vi "FAMM-FixPath.vi"(6 "path-IN":path, 8 "error in (no error)":errorcluster, 11 "FAMM in":T1={"FAMM_PAQ_Layers"=0, "FAMM_PAQ_resolution"=0.0, "PAQ_TAGs"=[], "WAQ_TAGs"=[], "EAQ_TAGs"=[], "All_TAGs"=[], "PAQtagProps"=[], "WAQtagProps"=[], "EAQtagProps"=[], "DBAL_class"=refnum, "PAQ_memory"=[], "PAQupdates"=[], "FAMM_Size"={"other"=0, "1day"=0, "1week"=0}, "DatabaseFileExtention"="", "DatabaseSaveRate"=0.0, "Database_path"=path "G:/Sgraph_database", "DBAL-Queue"=refnum, "OS_name"="undefined"} {"FAMM_Size"."1week" format="%.0p"; "FAMM_Size"."1day" format="%.0p"; "FAMM_Size"."other" format="%.0p"; "EAQtagProps"."TagFunc" format="%08x"; "EAQtagProps"."RangeL" format="%.2f"; "EAQtagProps"."RangeH" format="%.2f"; "WAQtagProps"."TagFunc" format="%08x"; "WAQtagProps"."RangeL" format="%.2f"; "WAQtagProps"."RangeH" format="%.2f"; "PAQtagProps"."TagFunc" format="%08x"; "PAQtagProps"."RangeL" format="%.2f"; "PAQtagProps"."RangeH" format="%.2f"; "FAMM_PAQ_resolution" format="%.1p"}) -> (0 "error out":errorcluster, 3 "FAMM out":T1={"FAMM_PAQ_Layers"=0, "FAMM_PAQ_resolution"=0.0, "PAQ_TAGs"=[], "WAQ_TAGs"=[], "EAQ_TAGs"=[], "All_TAGs"=[], "PAQtagProps"=[], "WAQtagProps"=[], "EAQtagProps"=[], "DBAL_class"=refnum, "PAQ_memory"=[], "PAQupdates"=[], "FAMM_Size"={"other"=0, "1day"=0, "1week"=0}, "DatabaseFileExtention"="", "DatabaseSaveRate"=0.0, "Database_path"=path "G:/Sgraph_database", "DBAL-Queue"=refnum, "OS_name"="undefined"} {"FAMM_Size"."1week" format="%.0p"; "FAMM_Size"."1day" format="%.0p"; "FAMM_Size"."other" format="%.0p"; "EAQtagProps"."TagFunc" format="%08x"; "EAQtagProps"."RangeL" format="%.2f"; "EAQtagProps"."RangeH" format="%.2f"; "WAQtagProps"."TagFunc" format="%08x"; "WAQtagProps"."RangeL" format="%.2f"; "WAQtagProps"."RangeH" format="%.2f"; "PAQtagProps"."TagFunc" format="%08x"; "PAQtagProps"."RangeL" format="%.2f"; "PAQtagProps"."RangeH" format="%.2f"; "FAMM_PAQ_resolution" format="%.1p"}, 4 "path-OUT":path)   [LabVIEW 2020, in "Sgraph_lib_V1.lvlib" / "FAMM.lvclass"]
doc: "Fix the OS dependency of a file path.\nUnix path definitions (Mac and Linux) differ from Windows type path definitions and therefore need to be adapted."
uses:
  FAMM.lvclass
  controls/FAMM-attributes.ctl
  Common/controls/typedef_com_TagProp.ctl
  DBAL/DBAL.lvclass
  PAQ-memory.lvclass
  DBAL/controls/DBAL_Command.ctl
  DBAL/controls/DBAL-commands.ctl
  Builds/Sgraph_lib_V1.lvlib
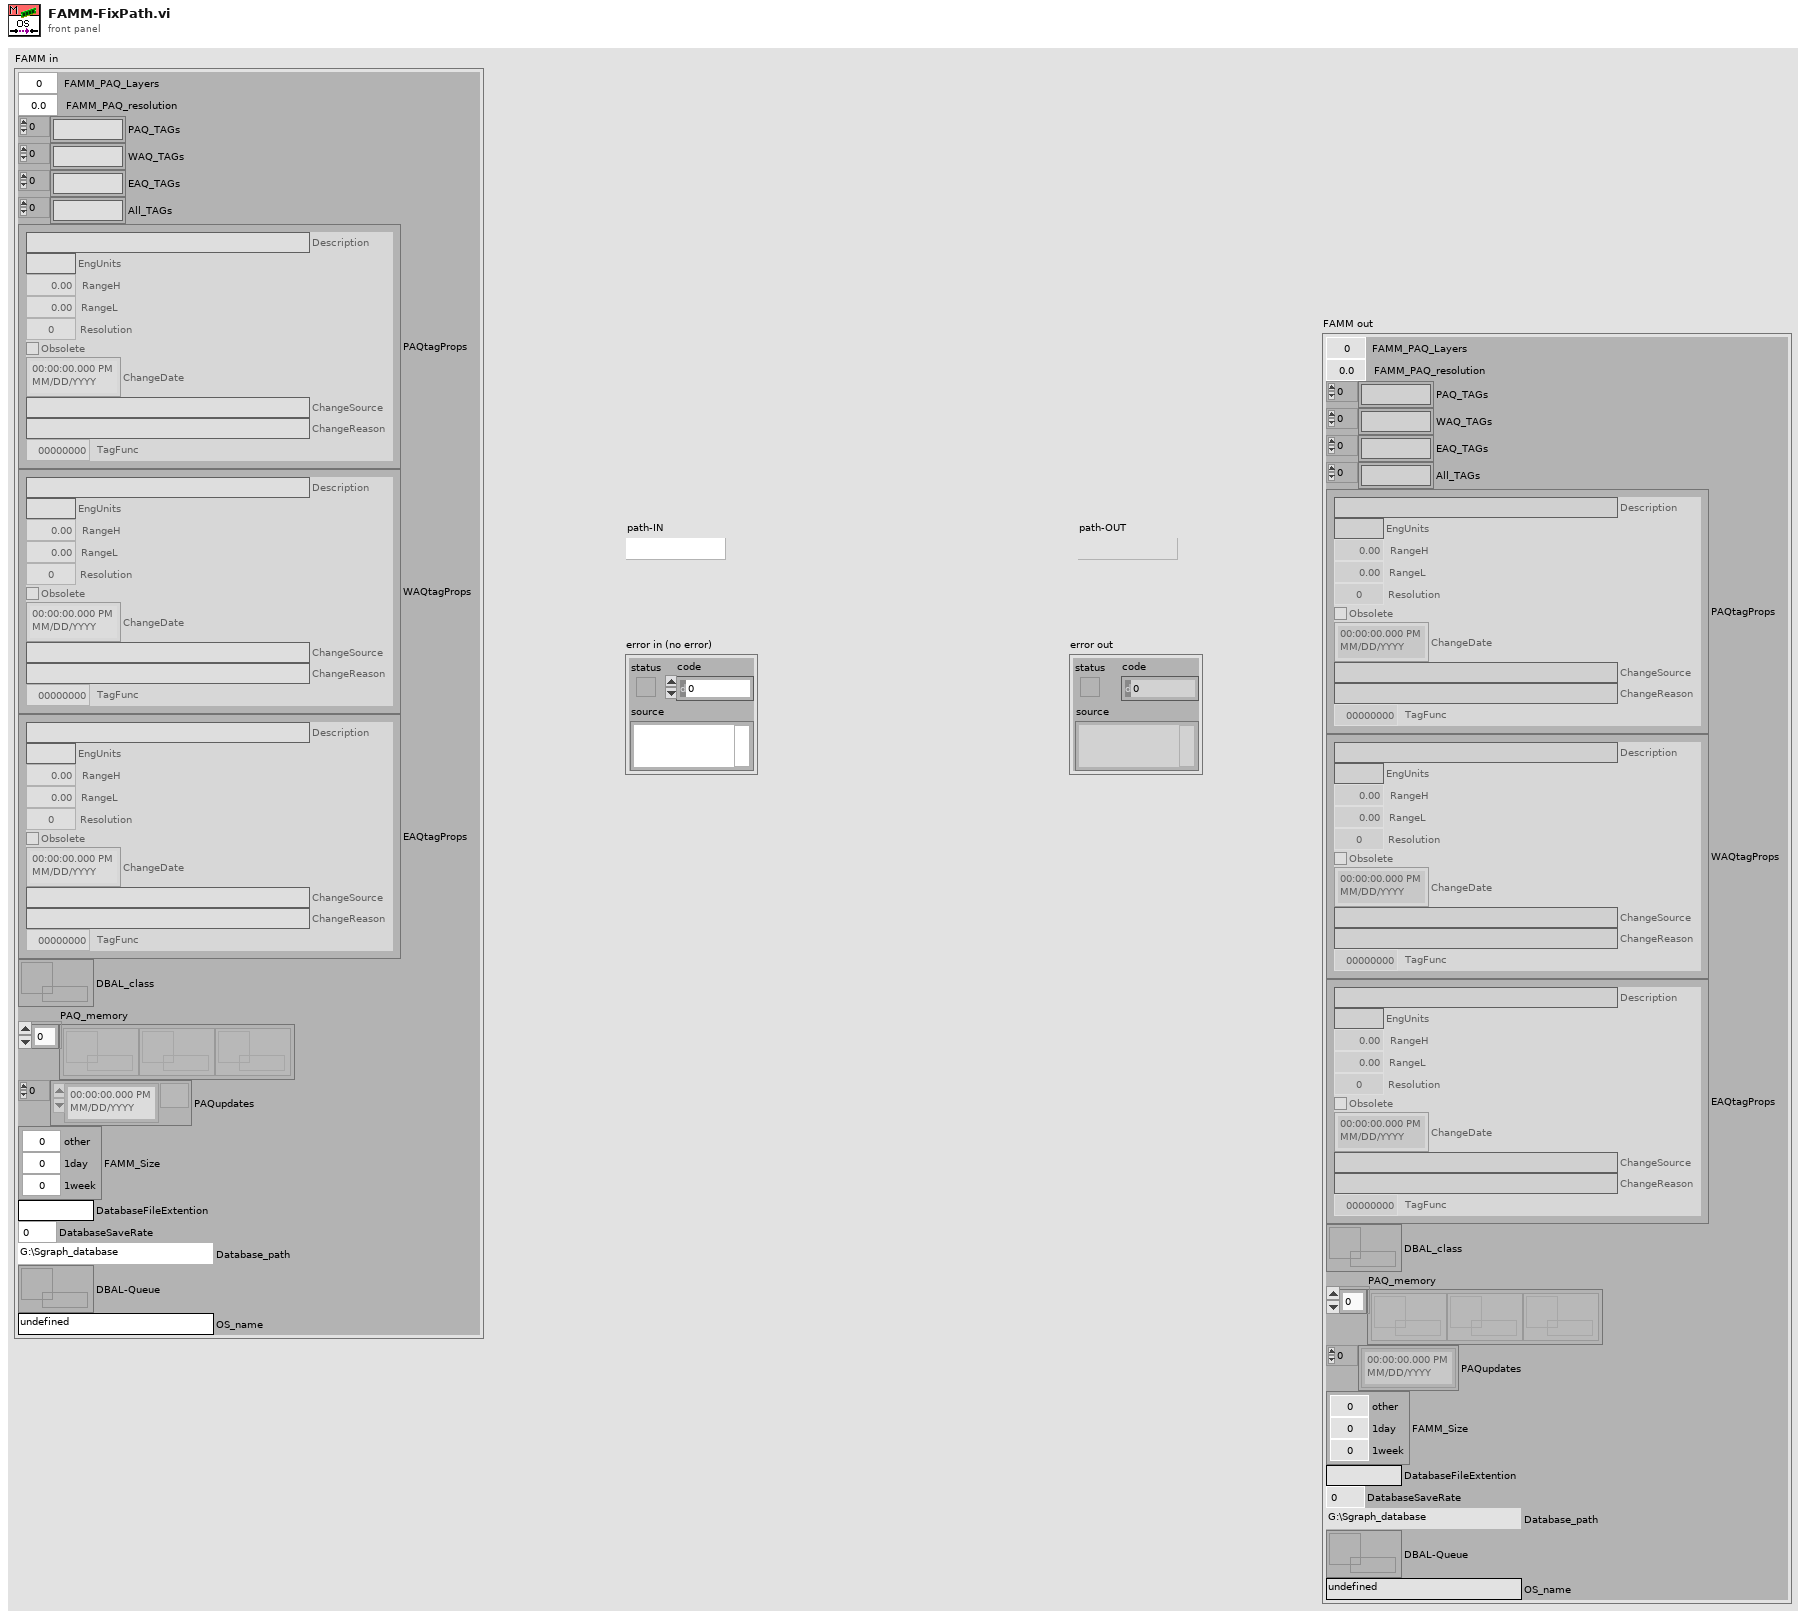
[diagram p1: front panel]
types:
  T1 = typedef "Sgraph_lib_V1.lvlib/FAMM.lvclass/FAMM-attributes.ctl" = cluster{"FAMM_PAQ_Layers":i32, "FAMM_PAQ_resolution":dbl, "PAQ_TAGs":string[], "WAQ_TAGs":string[], "EAQ_TAGs":string[], "All_TAGs":string[], "PAQtagProps":T2[], "WAQtagProps":T2[], "EAQtagProps":T2[], "DBAL_class":refnum<data-value>, "PAQ_memory":refnum<data-value>[], "PAQupdates":timestamp[], "FAMM_Size":cluster{"other":i32, "1day":i32, "1week":i32}, "DatabaseFileExtention":string, "DatabaseSaveRate":dbl, "Database_path":path, "DBAL-Queue":refnum<queue>, "OS_name":string}
  T2 = typedef "Sgraph_lib_V1.lvlib/typedef_com_TagProp.ctl" = cluster{"Description":string, "EngUnits":string, "RangeH":dbl, "RangeL":dbl, "Resolution":i32, "Obsolete":bool, "ChangeDate":timestamp, "ChangeSource":string, "ChangeReason":string, "TagFunc":u32}
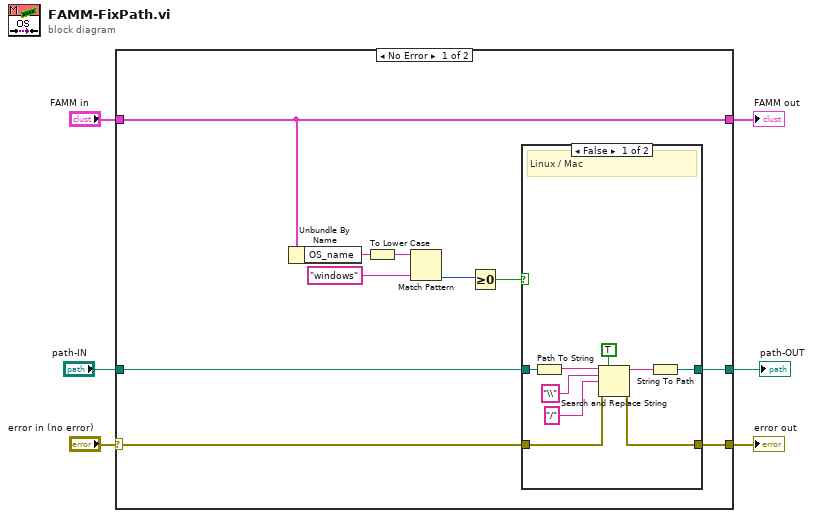
[diagram p0: block diagram]
diagram:
  n1 = case shown="No Error" "error in (no error)" {
    selector: "error in (no error)" -> [w13 w30]
    tunnel: [w12 w30] -> w5
    tunnel: [w7 w29] -> w3
    tunnel: "FAMM in" -> [w7 w29]
    tunnel: "path-IN" -> [w15 w28]
    tunnel: [w14 w28] -> w1
    frame No Error {
      n2 = Unbundle By Name(w7) -> ("OS_name"=w11:string)
      n3 = To Lower Case(string=w11) -> (all lower case string=w10:string)
      n4 = Match Pattern(string=w10, regular expression="windows") -> (offset past match=w8:i32)  [unwired: 1 in, 3 out]
      n5 = Greater Or Equal To 0?(x=w8) -> (x >= 0?=w16:bool)
      n6 = case shown="False" w16 {
        tunnel: w15 -> [w25 w27]
        tunnel: [w17 w27] -> w14
        tunnel: w13 -> [w20 w26]
        tunnel: [w19 w26] -> w12
        frame False {
          # "Linux / Mac"
          n7 = Path To String(path=w25) -> (string=w24:string)
          n8 = Search and Replace String(replace all?=TRUE ("replace all? (F)"), input string=w24, search string="\\", replace string="/", error in=w20) -> (result string=w18:string, error out=w19:errorcluster)  [unwired: 3 in, 2 out]
          n9 = String To Path(string=w18) -> (path=w17:path)
        }
        frame True {
          # "Windows"
        }
      }
    }
    frame Error {
    }
  }
  "error out" <- w5
  "FAMM out" <- w3
  "path-OUT" <- w1
